vi "Subpanel UI.vi"(8 "error in (no error)":errorcluster, 10 "Message Queue":refnum<queue>, 11 "Temperature Controller in":refnum<class "Temperature Controller.lvclass">) -> (0 "error out":errorcluster, 3 "Temperature Controller out":refnum<class "Temperature Controller.lvclass">)   [LabVIEW 2020, in "Temperature Controller.lvclass"]
doc: "Data display subpanel associated with the Temperature Controller class."
uses:
  Temperature Controller.lvclass
  Temperature Controller.lvclass/Temperature Controller.ctl
  Sub VIs/Message Queue/test Message Queue.lvlib
  <vilib>/ErrorRing/Error Ring.xnode
  <vilib>/Utility/error.llb/Error Cluster From Error Code.vi
  Sub VIs/Message Queue/Enqueue Message (Single).vi
  Sub VIs/Message Queue/Message Cluster.ctl
panel:
  out "Name":string
  out "Running?":bool
  in  "Time Interval (sec)":i32=1200
  out "Temperature Graph":cluster{timestamp[], dbl[]}[](graph)
  out "Current Temperature (C)":dbl format="%.3g"
  out "Setpoint (C)":dbl format="%.3f"
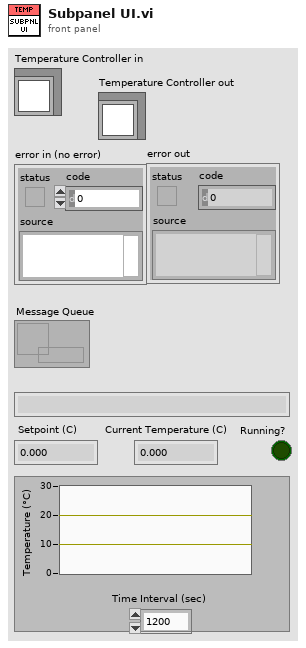
[diagram p1: front panel]
types:
  T1 = cluster{"Data Timestamps":timestamp[], "Data Values":dbl[], "Setpoint":dbl[], "Previous Run State":bool}
  T2 = typedef "Temperature Controller.lvclass/Temperature Controller State.ctl" = cluster{"VISA Resource":refnum<visa-resource-name>, "Setpoint":dbl, "Running":bool, "Running Since":timestamp, "Data Point":cluster{"Time Stamp":timestamp, "Value":dbl}, "Sample Rate (sec/sample)":dbl}
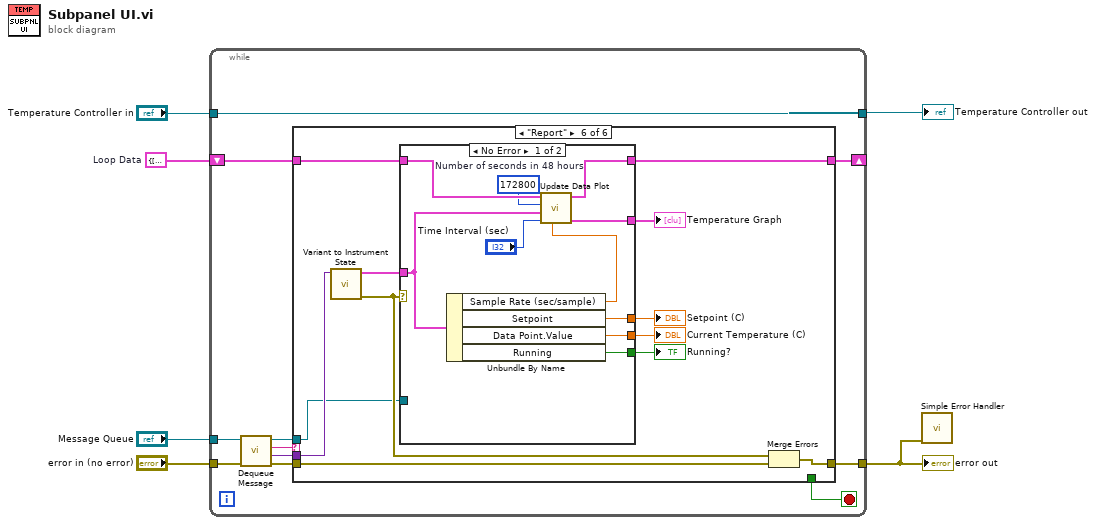
[diagram p0: block diagram]
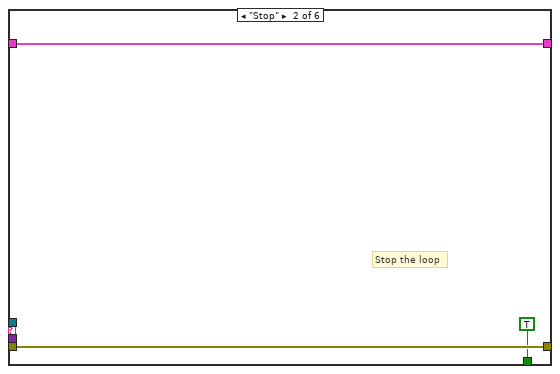
[diagram p3: hidden frame]
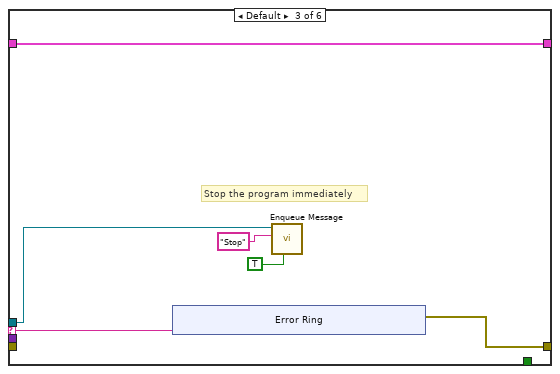
[diagram p4: hidden frame]
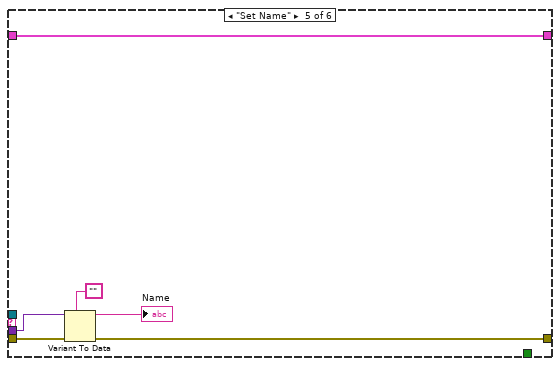
[diagram p6: hidden frame]
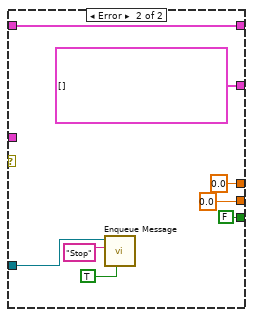
[diagram p7: hidden frame]
diagram:
  w1 = T1 {"Data Timestamps"=[], "Data Values"=[], "Setpoint"=[], "Previous Run State"=FALSE}  # Loop Data
  n1 = while {
    tunnel: [w7] -> w5
    tunnel: "Temperature Controller in" -> [w7]
    tunnel: [w11] -> w2
    tunnel: "error in (no error)" -> [w17]
    tunnel: "Message Queue" -> [w16]
    shift-right: [w9] -> _
    shift-left: w1 -> [w8]
    stop <- w10 stop-if-true
    n2 = call "Dequeue Message.vi"("error in (no error)"=w17, "Message Queue"=w16) -> ("error out"=w12:errorcluster, "Message Data"=w14:variant, "Message"=w15:string, "dup Message Queue"=w13:refnum<queue>)  [unwired: 6 in]
    n3 = case shown="\"Report\"" w15 {
      selector: w15 -> [_ _ w27 _ _ _]
      tunnel: w14 -> [_ _ _ _ w42 w51]
      tunnel: w13 -> [_ _ w25 _ _ w44]
      tunnel: w12 -> [w18 w22 _ w37 w41 w55]
      tunnel: [w18 w22 w26 w37 w40 w46] -> w11
      tunnel: [_ TRUE _ _ _ _] -> w10
      tunnel: [w19 w20 w28 w36 w43 w53] -> w9
      tunnel: w8 -> [w19 w20 w28 w36 w43 w54]
      frame "Initialize" {
      }
      frame "Stop" {
        # "Stop the loop"
      }
      frame Default {
        # "Stop the program immediately"
        n4 = xnode "Error Ring"("parameter 0"=w27) -> ("error out"=w26:errorcluster)
        n5 = call-poly "Enqueue Message.vi"("Priority Message? (F)"=TRUE, "Message"="Stop", "Message Queue"=w25) -> ()  [unwired: 7 in, 2 out]
      }
      frame "--- Copy this frame ---" {
      }
      frame "Set Name" {
        n6 = Variant To Data(error in=w41, type="", Variant=w42) -> (data=→"Name":string, error out=w40:errorcluster)
      }
      frame "Report" {
        n7 = call "Variant to Instrument State.vi"("Message Data"=w51) -> ("error out"=w45:errorcluster, "Instrument State"=w50:T2)  [unwired: 9 in]
        n8 = case shown="No Error" w45 {
          tunnel: w54 -> [w65 w73]
          tunnel: [w64 w73] -> w53
          tunnel: [w63 cluster{timestamp[], dbl[]}[] [] ("Updated Plot History")] -> w52
          tunnel: w50 -> [w62 _]
          tunnel: [w60 0.0 ("Setpoint")] -> w49
          tunnel: [w59 0.0 ("Current Temperature")] -> w48
          tunnel: [w58 FALSE ("Running")] -> w47
          tunnel: w44 -> [_ w68]
          frame No Error {
            w56 = 172800  # Number of seconds in 48 hours
            n9 = Unbundle By Name(w62) -> ("Sample Rate (sec/sample)"=w57:dbl, "Setpoint"=w60:dbl, "Data Point.Value"=w59:dbl, "Running"=w58:bool)
            n10 = call "Update Data Plot.vi"("Sample Rate (sec/sample)"=w57, "Time interval (s)"="Time Interval (sec)", "Temperature Controller State"=w62, "History length"=w56, "Graph History Arrays in"=w65) -> ("Updated Plot History"=w63:cluster{timestamp[], dbl[]}[], "Graph History Arrays out"=w64:T1)  [unwired: 5 in]
          }
          frame Error {
            n11 = call-poly "Enqueue Message.vi"("Priority Message? (F)"=TRUE, "Message"="Stop", "Message Queue"=w68) -> ()  [unwired: 7 in, 2 out]
          }
        }
        "Setpoint (C)" <- w49
        "Temperature Graph" <- w52
        "Running?" <- w47
        "Current Temperature (C)" <- w48
        n12 = Merge Errors(w45, w55) -> (w46:errorcluster)
      }
    }
  }
  "error out" <- w2
  "Temperature Controller out" <- w5
  n13 = call <vilib>:"Simple Error Handler.vi"("error in (no error)"=w2) -> ()  [unwired: 4 in, 5 out]
